vi "Flashing.vi"(11 "Error":bool) -> (3 "Light":bool)   [LabVIEW 2013]
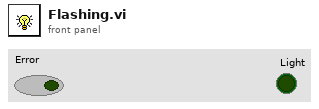
[diagram p1: front panel]
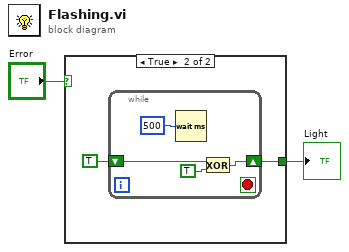
[diagram p0: block diagram]
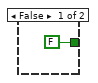
[diagram p2: hidden frame]
diagram:
  n1 = case shown="True" "Error" {
    tunnel: [FALSE w5] -> w1
    frame False {
    }
    frame True {
      n2 = while {
        shift-right: [w6] -> w5
        shift-left: TRUE -> [w7]
        stop <- _ stop-if-true
        n3 = Wait (ms)(milliseconds to wait=u32 500) -> ()  [unwired: 1 out]
        n4 = Exclusive Or(1:TRUE, 2:w7) -> (0:w6:bool)
      }
    }
  }
  "Light" <- w1
